vi "_Remote Calculate ADC.vi"(4 "ADC Table":T1[](array[typedef]), 5 "Unit":bool, 6 "ADC Channel (64)":u8, 7 "ADC Values":i32[](array[numeric])) -> (1 "In Range?":bool, 2 "User Value":dbl, 3 "Raw Reading":dbl)   [LabVIEW 2012]
uses:
  Type/_RT Configuration 2.ctl
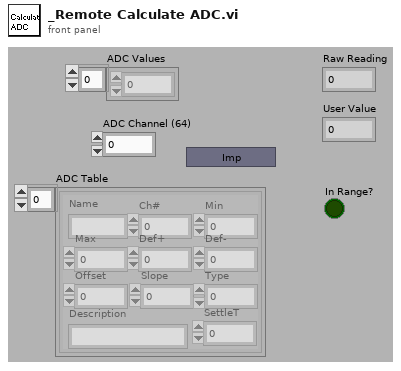
[diagram p1: front panel]
types:
  T1 = typedef "_RT Configuration 2.ctl" = cluster{"Name":string, "Ch#":u8, "Min":dbl, "Max":dbl, "Def+":dbl, "Def-":dbl, "Offset":dbl, "Slope":dbl, "Type":u8, "Description":string, "SettleT":dbl}
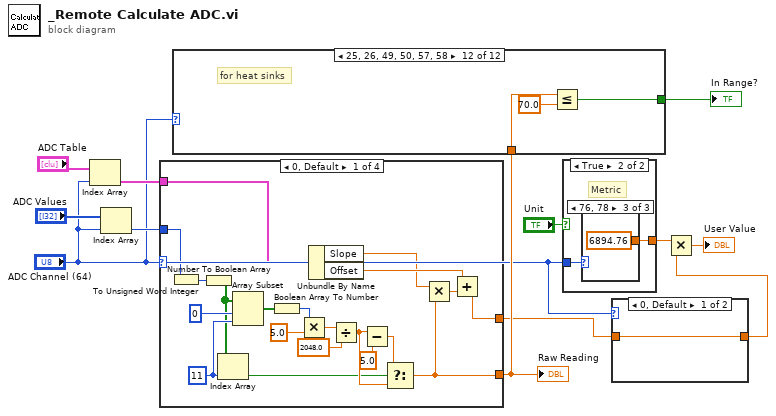
[diagram p0: block diagram]
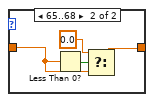
[diagram p2: hidden frame]
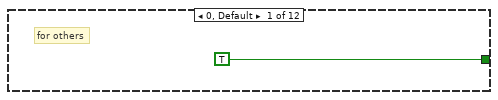
[diagram p3: hidden frame]
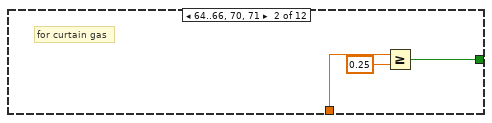
[diagram p4: hidden frame]
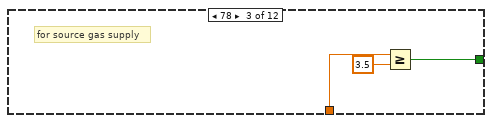
[diagram p5: hidden frame]
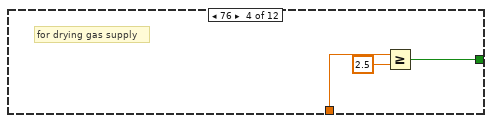
[diagram p6: hidden frame]
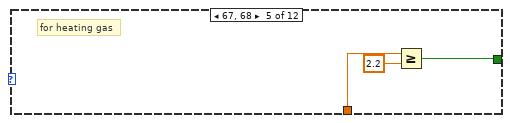
[diagram p7: hidden frame]
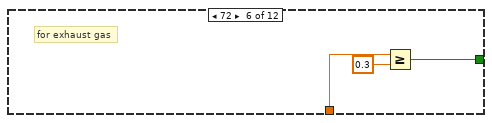
[diagram p8: hidden frame]
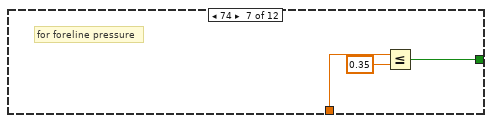
[diagram p9: hidden frame]
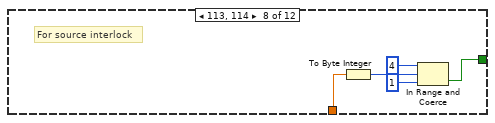
[diagram p10: hidden frame]
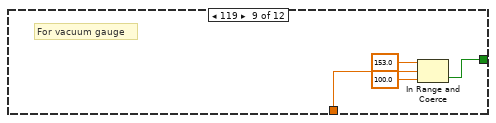
[diagram p11: hidden frame]
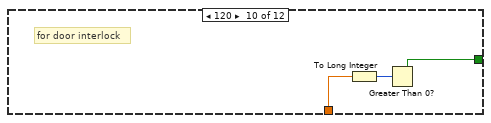
[diagram p12: hidden frame]
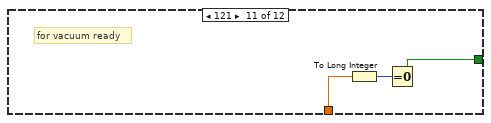
[diagram p13: hidden frame]
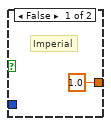
[diagram p14: hidden frame]
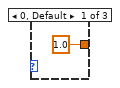
[diagram p15: hidden frame]
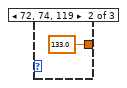
[diagram p16: hidden frame]
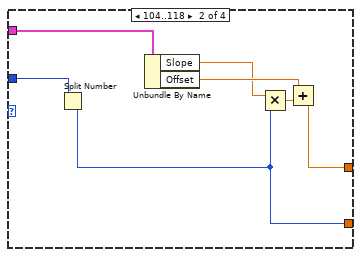
[diagram p17: hidden frame]
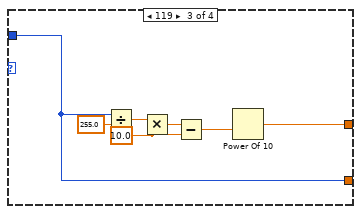
[diagram p18: hidden frame]
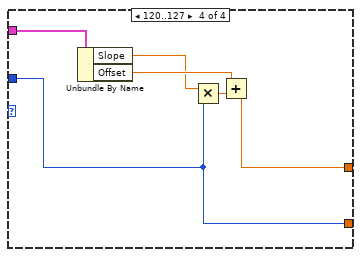
[diagram p19: hidden frame]
diagram:
  n1 = Index Array(array="ADC Table", index="ADC Channel (64)") -> (element=w9:T1)
  n2 = Index Array(array="ADC Values", index="ADC Channel (64)") -> (element=w11:i32)
  n3 = case shown="0, Default" "ADC Channel (64)" {
    tunnel: [w15 w34 w40 w48] -> w4
    tunnel: w11 -> [w19 w39 w40 w48]
    tunnel: [w13 w33 w41 w47] -> w2
    tunnel: w9 -> [w14 w35 _ w49]
    frame 0, Default {
      w21 = 11 ("index")
      n4 = To Unsigned Word Integer(number=w19) -> (unsigned 16bit integer=w29:u16)
      n5 = Number To Boolean Array(number=w29) -> (Boolean array=w20:bool[])
      n6 = Index Array(array=w20, index=w21) -> (element=w26:bool)
      n7 = Array Subset(array=w20, index=0, length=w21) -> (w22:bool[])
      n8 = Boolean Array To Number(Boolean array=w22) -> (number=w25:u32)
      n9 = Multiply(x=w25, y=5.0) -> (x*y=w30:dbl)
      n10 = Unbundle By Name(w14) -> ("Slope"=w16:dbl, "Offset"=w17:dbl)
      n11 = Divide(x=w30, y=2048.0) -> (x/y=w32:dbl)
      n12 = Subtract(x=w32, y=5.0) -> (x-y=w28:dbl)
      n13 = Select(t=w28, s=w26, f=w32) -> (s? t:f=w15:dbl)
      n14 = Multiply(x=w16, y=w15) -> (x*y=w18:dbl)
      n15 = Add(x=w17, y=w18) -> (x+y=w13:dbl)
    }
    frame 104..118 {
      n16 = Split Number(x=w39) -> (lo(x)=w34:u16)  [unwired: 1 out]
      n17 = Unbundle By Name(w35) -> ("Slope"=w36:dbl, "Offset"=w37:dbl)
      n18 = Multiply(x=w36, y=w34) -> (x*y=w38:dbl)
      n19 = Add(x=w37, y=w38) -> (x+y=w33:dbl)
    }
    frame 119 {
      w42 = sgl 10.0 ("y")
      n20 = Divide(x=w40, y=sgl 255.0) -> (x/y=w45:sgl)
      n21 = Multiply(x=w45, y=w42) -> (x*y=w44:sgl)
      n22 = Subtract(x=w44, y=w42) -> (x-y=w43:sgl)
      n23 = Power Of 10(x=w43) -> (10^x=w41:sgl)
    }
    frame 120..127 {
      n24 = Unbundle By Name(w49) -> ("Slope"=w50:dbl, "Offset"=w51:dbl)
      n25 = Multiply(x=w50, y=w48) -> (x*y=w52:dbl)
      n26 = Add(x=w51, y=w52) -> (x+y=w47:dbl)
    }
  }
  "Raw Reading" <- w4
  n27 = case shown="25, 26, 49, 50, 57, 58" "ADC Channel (64)" {
    tunnel: [TRUE w54 w57 w60 w64 w66 w69 w72 w77 w81 w84 w87] -> w8
    tunnel: w4 -> [_ w56 w59 w62 w65 w68 w71 w76 w78 w82 w85 w89]
    frame 0, Default {
      # "for others"
    }
    frame 64..66, 70, 71 {
      # "for curtain gas"
      n28 = Greater Or Equal?(x=w56, y=0.25) -> (x >= y?=w54:bool)
    }
    frame 78 {
      # "for source gas supply"
      n29 = Greater Or Equal?(x=w59, y=3.5) -> (x >= y?=w57:bool)
    }
    frame 76 {
      # "for drying gas supply"
      n30 = Greater Or Equal?(x=w62, y=2.5) -> (x >= y?=w60:bool)
    }
    frame 67, 68 {
      # "for heating gas"
      n31 = Greater Or Equal?(x=w65, y=2.2) -> (x >= y?=w64:bool)
    }
    frame 72 {
      # "for exhaust gas"
      n32 = Greater Or Equal?(x=w68, y=0.3) -> (x >= y?=w66:bool)
    }
    frame 74 {
      # "for foreline pressure"
      n33 = Less Or Equal?(x=w71, y=0.35) -> (x <= y?=w69:bool)
    }
    frame 113, 114 {
      # "For source interlock"
      n34 = To Byte Integer(number=w76) -> (8bit integer=w73:i8)
      n35 = In Range and Coerce(upper limit=i8 4, x=w73, lower limit=i8 1) -> (In Range?=w72:bool)  [unwired: 1 out]
    }
    frame 119 {
      # "For vacuum gauge"
      n36 = In Range and Coerce(upper limit=sgl 153.0, x=w78, lower limit=sgl 100.0) -> (In Range?=w77:bool)  [unwired: 1 out]
    }
    frame 120 {
      # "for door interlock"
      n37 = To Long Integer(number=w82) -> (32bit integer=w83:i32)
      n38 = Greater Than 0?(x=w83) -> (x > 0?=w81:bool)
    }
    frame 121 {
      # "for vacuum ready"
      n39 = To Long Integer(number=w85) -> (32bit integer=w86:i32)
      n40 = Equal To 0?(x=w86) -> (x = 0?=w84:bool)
    }
    frame 25, 26, 49, 50, 57, 58 {
      # "for heat sinks"
      n41 = Less Or Equal?(x=w89, y=70.0) -> (x <= y?=w87:bool)
    }
  }
  "In Range?" <- w8
  n42 = case shown="True" "Unit" {
    tunnel: "ADC Channel (64)" -> [_ w92]
    tunnel: [1.0 w91] -> w6
    frame False {
      # "Imperial"
    }
    frame True {
      # "Metric"
      n43 = case shown="76, 78" w92 {
        tunnel: [1.0 133.0 6894.76] -> w91
        frame 0, Default {
        }
        frame 72, 74, 119 {
        }
        frame 76, 78 {
        }
      }
    }
  }
  n44 = case shown="0, Default" "ADC Channel (64)" {
    tunnel: [w96 w99] -> w1
    tunnel: w2 -> [w96 w98]
    frame 0, Default {
    }
    frame 65..68 {
      n45 = Less Than 0?(x=w98) -> (x < 0?=w100:bool)
      n46 = Select(t=0.0, s=w100, f=w98) -> (s? t:f=w99:dbl)
    }
  }
  n47 = Multiply(x=w6, y=w1) -> (x*y=→"User Value":dbl)
